vi "fgv_cpu-mem_data.vi"(7 "cmd":T1, 10 "memory":dbl, 11 "cpu":dbl) -> (2 "memory out":dbl, 3 "cpu out":dbl)   [LabVIEW 2019]
uses:
  Ctrl/cmd_common.ctl
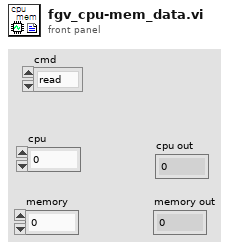
[diagram p1: front panel]
types:
  T1 = typedef "cmd_common.ctl" = enum16{"read", "write"}
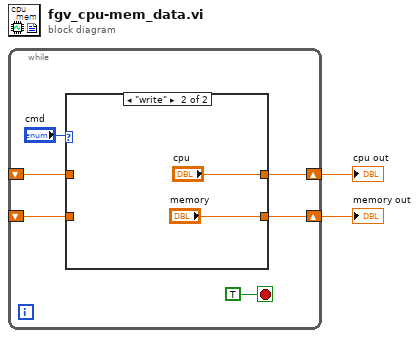
[diagram p0: block diagram]
diagram:
  n1 = while {
    shift-right: [w5] -> w2
    shift-left: _ -> [w4]
    shift-right: [w6] -> w1
    shift-left: _ -> [w3]
    stop <- TRUE stop-if-true
    n2 = case shown="\"write\"" "cmd" {
      tunnel: [w9 "memory"] -> w6
      tunnel: [w10 "cpu"] -> w5
      tunnel: w4 -> [w10 _]
      tunnel: w3 -> [w9 _]
      frame "read", Default {
      }
      frame "write" {
      }
    }
  }
  "cpu out" <- w2
  "memory out" <- w1
